vi "test_1.vi"() -> ()   [LabVIEW 2010]
panel:
  out "布尔 16":bool
  out "布尔 15":bool
  out "布尔 14":bool
  out "布尔 13":bool
  out "布尔 12":bool
  out "布尔 11":bool
  out "布尔 10":bool
  out "布尔 9":bool
  out "布尔 8":bool
  out "布尔 7":bool
  out "布尔 6":bool
  out "布尔 5":bool
  out "布尔 4":bool
  out "布尔 3":bool
  out "布尔 2":bool
  out "布尔":bool
  out "合格":bool
  in  "输入值":enum16{"0", "1"}[](array[ring])
  in  "是否选择":bool[](array[boolean])
  in  "反馈值":bool[](array[boolean])
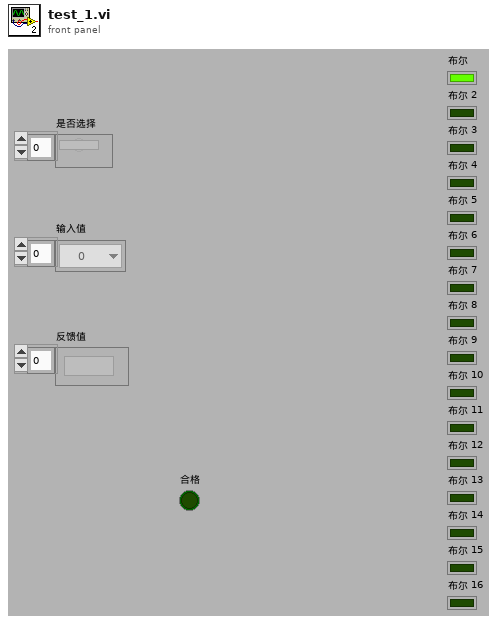
[diagram p1: front panel]
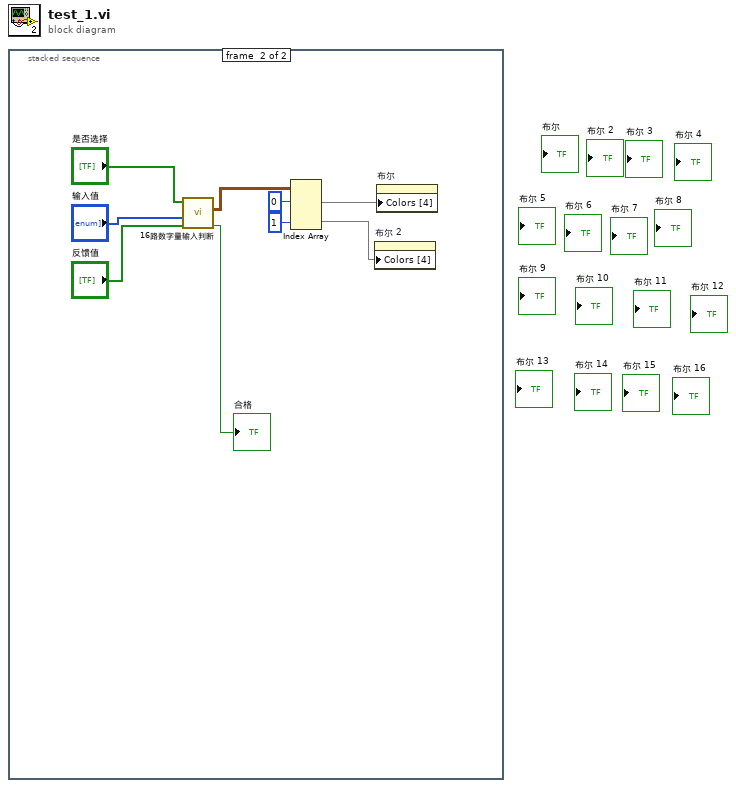
[diagram p0: block diagram]
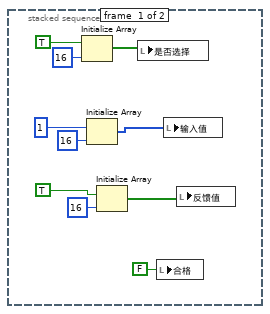
[diagram p2: hidden frame]
diagram:
  n1 = stacked-sequence {
    frame #0 {
      n2 = Initialize Array(TRUE, 16 ("维数大小")) -> (w8:bool[])
      n3 = Initialize Array(u16 1, 16 ("维数大小")) -> (w5:u16[])
      n4 = Initialize Array(TRUE, 16 ("维数大小")) -> (w2:bool[])
      n5 = local write "是否选择"(w8) -> ()
      n6 = local write "合格"(FALSE ("合格")) -> ()
      n7 = local write "输入值"(w5) -> ()
      n8 = local write "反馈值"(w2) -> ()
    }
    frame #1 {
      n9 = call "16路数字量输入判断.vi"("反馈值"="反馈值", "输入值"="输入值", "是否选择"="是否选择") -> ("合格"=→"合格":bool, "结果"=w15:cluster{u32, u32}[][])  [unwired: 6 in, 1 out]
      n10 = Index Array(array=w15, index (row) #1=0 ("索引 (行)"), index (row) #2=1 ("索引 (行)")) -> (element #1=w13:cluster{u32, u32}[], element #2=w11:cluster{u32, u32}[])  [unwired: 2 in]
      n11 = property on="布尔 2" class="Bool (严格)"("Colors [4]"=w11) -> ()  [unwired: 2 in, 2 out]
      n12 = property on="布尔" class="Bool (严格)"("Colors [4]"=w13) -> ()  [unwired: 2 in, 2 out]
    }
  }
